vi "UMLEditor_AggregationClusterDialogControl.vi"(0 "Position":T2, 1 "OK-Button":refnum<vi>, 2 "Cancel-Button":refnum<vi>, 3 "String":refnum<vi>, 4 "Cluster":refnum<vi>, 5 "error in (no error)":errorcluster, 6 "Action(SelectSelect)":T3(ring), 7 "screenRef":refnum<vi>, 9 "StartEndNodesIn":T1) -> (13 "StartEndNodes":T1, 15 "AddAggregate?":bool, 19 "error out":errorcluster)   [LabVIEW 2014]
doc: "Gets current diagram values"
uses:
  <resource>/Framework/Providers/Open_GDS/UML/UMLEditor/UMLEditor ClassToolButtons.ctl
  <vilib>/Utility/miscctls.llb/LVPositionTypeDef.ctl
  <resource>/Framework/Providers/Open_GDS/UML/AbstractNode_class/AbstractNode.lvclass
  <vilib>/Utility/miscctls.llb/LVPoint32TypeDef.ctl
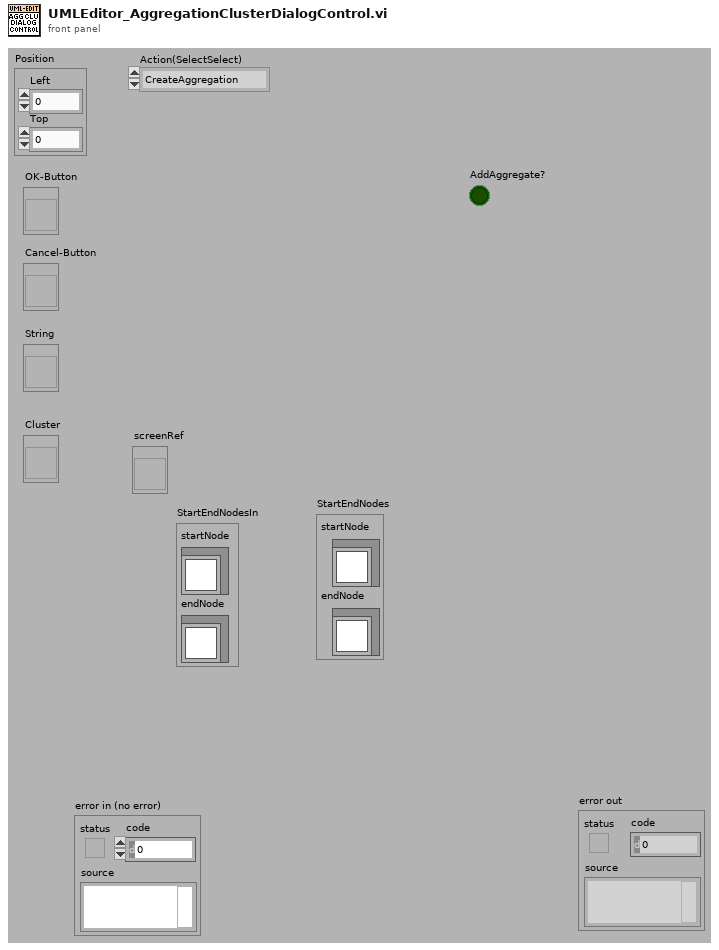
[diagram p1: front panel]
types:
  T1 = cluster{"startNode":refnum<class "AbstractNode.lvclass">, "endNode":refnum<class "AbstractNode.lvclass">}
  T2 = typedef "LVPositionTypeDef.ctl" = cluster{"Left":i32, "Top":i32}
  T3 = enum16{"CreateAggregation", "DeleteAggregation", "SetReferneces", "HideCluster", "GetStatus"}
  T4 = typedef "LVPoint32TypeDef.ctl" = cluster{"Horizontal":i32, "Vertical":i32}
  T5 = typedef "LVBoundsTypeDef.ctl" = cluster{"Width":u32, "Height":u32}
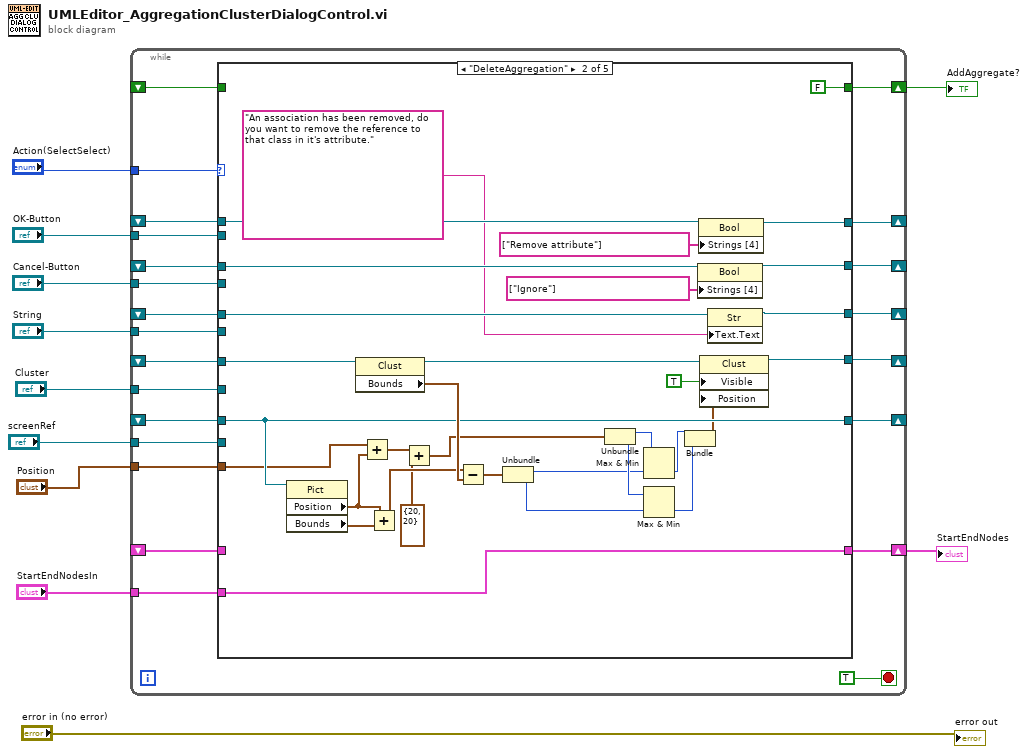
[diagram p0: block diagram]
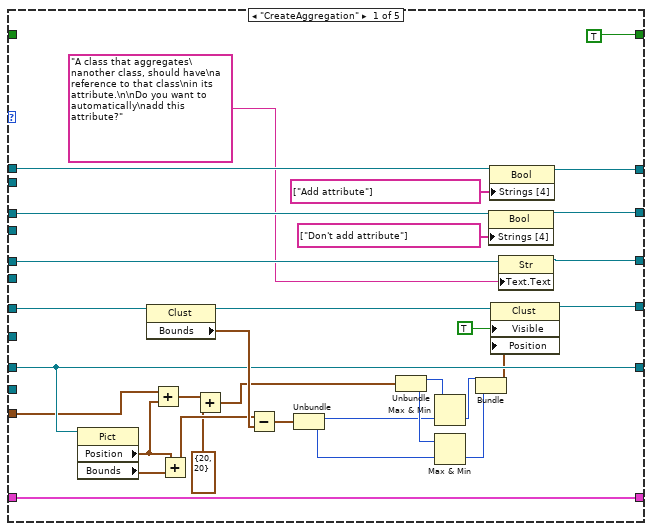
[diagram p2: hidden frame]
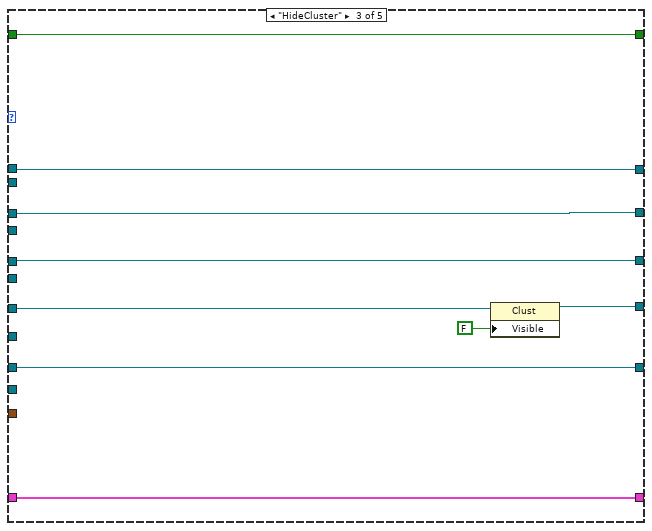
[diagram p3: hidden frame]
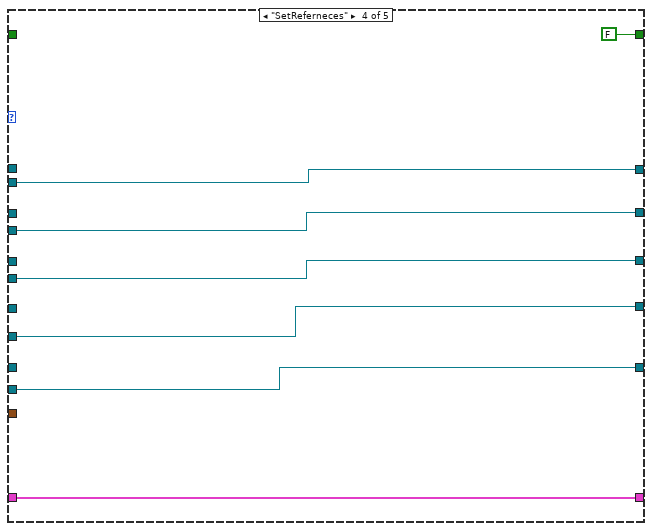
[diagram p4: hidden frame]
diagram:
  n1 = while {
    tunnel: "Action(SelectSelect)" -> [w34]
    shift-right: [w31] -> _
    shift-left: _ -> [w32]
    shift-right: [w29] -> _
    shift-left: _ -> [w30]
    shift-right: [w26] -> _
    shift-left: _ -> [w28]
    shift-right: [w25] -> _
    shift-left: _ -> [w27]
    tunnel: "OK-Button" -> [w24]
    tunnel: "Cancel-Button" -> [w23]
    tunnel: "String" -> [w22]
    tunnel: "Cluster" -> [w21]
    shift-right: [w20] -> _
    shift-left: _ -> [w18]
    tunnel: "screenRef" -> [w19]
    tunnel: "Position" -> [w17]
    shift-right: [w16] -> w3
    shift-left: _ -> [w15]
    shift-right: [w14] -> w1
    shift-left: _ -> [w12]
    tunnel: "StartEndNodesIn" -> [w13]
    stop <- TRUE stop-if-true
    n2 = case shown="\"DeleteAggregation\"" w34 {
      tunnel: w32 -> [w65 w97 w102 _ w121]
      tunnel: [w64 w96 w102 w114 w121] -> w31
      tunnel: w30 -> [w62 w94 w103 _ w120]
      tunnel: [w61 w93 w103 w113 w120] -> w29
      tunnel: w28 -> [w59 w91 w104 _ w119]
      tunnel: w27 -> [w43 w75 w107 _ w118]
      tunnel: [w58 w90 w104 w112 w119] -> w26
      tunnel: [w66 w98 w106 w111 w118] -> w25
      tunnel: w24 -> [_ _ _ w114 _]
      tunnel: w23 -> [_ _ _ w113 _]
      tunnel: w22 -> [_ _ _ w112 _]
      tunnel: w21 -> [_ _ _ w111 _]
      tunnel: [w45 w77 w101 w110 w117] -> w20
      tunnel: w19 -> [_ _ _ w110 _]
      tunnel: w18 -> [w45 w77 w101 _ w117]
      tunnel: w17 -> [w44 w76 _ _ _]
      tunnel: [TRUE FALSE w100 FALSE w116] -> w16
      tunnel: w15 -> [_ _ w100 _ w116]
      tunnel: [w35 w67 w99 w108 w115] -> w14
      tunnel: w13 -> [_ w67 _ _ _]
      tunnel: w12 -> [w35 _ w99 w108 w115]
      frame "CreateAggregation" {
        n3 = property on="Property Node" class="Pict"(reference=w45) -> ("Position"=w51:T2, "Bounds"=w53:T5)  [unwired: 1 in, 2 out]
        n4 = property on="Property Node" class="Clust"(reference=w43) -> (reference out=w42:refnum<vi>, "Bounds"=w55:T5)  [unwired: 1 in, 1 out]
        n5 = Add(x=w44, y=w51) -> (x+y=w50:T2)
        n6 = Add(x=w51, y=w53) -> (x+y=w52:T5)
        n7 = Add(x=w50, y=T4 {"Horizontal"=20, "Vertical"=20}) -> (x+y=w41:T2)
        n8 = Subtract(x=w52, y=w55) -> (x-y=w54:T5)
        n9 = Unbundle(w54) -> ("Width"=w40:u32, "Height"=w39:u32)
        n10 = Unbundle(w41) -> ("Left"=w48:i32, "Top"=w47:i32)
        n11 = Max & Min(x=w48, y=w40) -> (min(x,y)=w38:u32)  [unwired: 1 out]
        n12 = Max & Min(x=w47, y=w39) -> (min(x,y)=w46:u32)  [unwired: 1 out]
        n13 = Bundle(w38, w46) -> (w37:cluster{u32, u32})  [unwired: 1 out]
        n14 = property class="Bool"(reference=w62, "Strings [4]"=string[] ["Don't add attribute"]) -> (reference out=w61:refnum<vi>)  [unwired: 1 in, 1 out]
        n15 = property class="Bool"(reference=w65, "Strings [4]"=string[] ["Add attribute"]) -> (reference out=w64:refnum<vi>)  [unwired: 1 in, 1 out]
        n16 = property class="Clust"(reference=w42, "Visible"=TRUE, "Position"=w37) -> (reference out=w66:refnum<vi>)  [unwired: 1 in, 1 out]
        n17 = property class="Str"(reference=w59, "Text.Text"="A class that aggregates\nanother class, should have\na reference to that class\nin its attribute.\n\nDo you want to automatically\nadd this attribute?") -> (reference out=w58:refnum<vi>)  [unwired: 1 in, 1 out]
      }
      frame "DeleteAggregation" {
        n18 = property on="Property Node" class="Pict"(reference=w77) -> ("Position"=w83:T2, "Bounds"=w85:T5)  [unwired: 1 in, 2 out]
        n19 = property on="Property Node" class="Clust"(reference=w75) -> (reference out=w74:refnum<vi>, "Bounds"=w87:T5)  [unwired: 1 in, 1 out]
        n20 = Add(x=w76, y=w83) -> (x+y=w82:T2)
        n21 = Add(x=w83, y=w85) -> (x+y=w84:T5)
        n22 = Add(x=w82, y=T4 {"Horizontal"=20, "Vertical"=20}) -> (x+y=w73:T2)
        n23 = Subtract(x=w84, y=w87) -> (x-y=w86:T5)
        n24 = Unbundle(w86) -> ("Width"=w72:u32, "Height"=w71:u32)
        n25 = Unbundle(w73) -> ("Left"=w80:i32, "Top"=w79:i32)
        n26 = Max & Min(x=w80, y=w72) -> (min(x,y)=w70:u32)  [unwired: 1 out]
        n27 = Max & Min(x=w79, y=w71) -> (min(x,y)=w78:u32)  [unwired: 1 out]
        n28 = Bundle(w70, w78) -> (w69:cluster{u32, u32})  [unwired: 1 out]
        n29 = property class="Bool"(reference=w94, "Strings [4]"=string[] ["Ignore"]) -> (reference out=w93:refnum<vi>)  [unwired: 1 in, 1 out]
        n30 = property class="Bool"(reference=w97, "Strings [4]"=string[] ["Remove attribute"]) -> (reference out=w96:refnum<vi>)  [unwired: 1 in, 1 out]
        n31 = property class="Clust"(reference=w74, "Visible"=TRUE, "Position"=w69) -> (reference out=w98:refnum<vi>)  [unwired: 1 in, 1 out]
        n32 = property class="Str"(reference=w91, "Text.Text"="An association has been removed, do you want to remove the reference to that class in it's attribute.") -> (reference out=w90:refnum<vi>)  [unwired: 1 in, 1 out]
      }
      frame "HideCluster" {
        n33 = property class="Clust"(reference=w107, "Visible"=FALSE) -> (reference out=w106:refnum<vi>)  [unwired: 1 in, 1 out]
      }
      frame "SetReferneces" {
      }
      frame "GetStatus" {
      }
    }
  }
  "AddAggregate?" <- w3
  "StartEndNodes" <- w1
  "error out" <- "error in (no error)"
